vi "Exercise1.4-Accumulator_While.vi"() -> ()   [LabVIEW 2013]
panel:
  out "Sum":i32
  in  "N":i32
  out "Sum":i32
  in  "N":i32
  # "有问题"
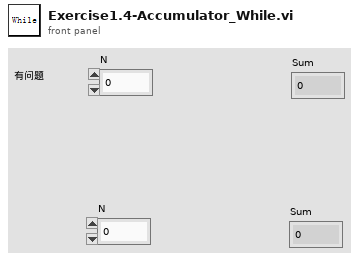
[diagram p1: front panel]
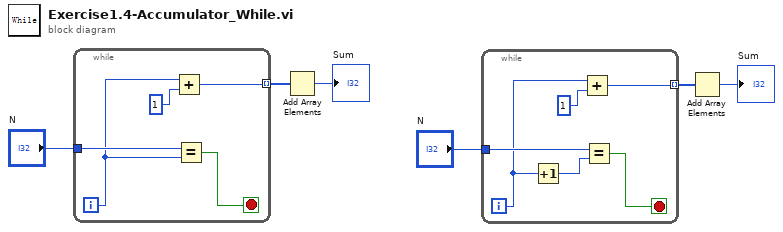
[diagram p0: block diagram]
diagram:
  n1 = while {
    tunnel: "N" -> [w8]
    tunnel: [w11] -> w1 mode=indexing
    i -> [w7]
    stop <- w9 stop-if-true
    n2 = Add(x=w7, y=1) -> (x+y=w11:i32)
    n3 = Equal?(x=w8, y=w7) -> (x = y?=w9:bool)
  }
  n4 = Add Array Elements(numeric array=w1) -> (sum=→"Sum":i32)
  n5 = while {
    tunnel: "N" -> [w14]
    tunnel: [w17] -> w4 mode=indexing
    i -> [w12]
    stop <- w15 stop-if-true
    n6 = Increment(x=w12) -> (x+1=w13:i32)
    n7 = Add(x=w12, y=1) -> (x+y=w17:i32)
    n8 = Equal?(x=w14, y=w13) -> (x = y?=w15:bool)
  }
  n9 = Add Array Elements(numeric array=w4) -> (sum=→"Sum":i32)
